vi "JoyStick_Global.vi"() -> ()   [LabVIEW 2015]
doc: "This global VI can contain as many global variables as you need. Place a control on the panel, give it a good name. To read or write to it from a VI, drag the icon to the diagram of that VI. You can also drag from the project. Click on the node to change which global you access. You shouldn't have multiple locations writing to a global or it will cause a race-condition."
uses:
  <vilib>/Rock Robotics/WPI/Camera/WPI_CameraImageSize.ctl
  <vilib>/Rock Robotics/WPI/DriverStation/WPI_DriverStationRobotMode2.ctl
panel:
  out "Intake_Sensor_LED":bool
  out "Stage_Sensor_LED":bool
  out "Light_Show":bool
  out "Low_Goal":bool
  in  "Climb_Speed":dbl
  in  "Climb_Pneu":bool
  in  "Auto_Aim":bool
  in  "Flipper_Man":bool
  in  "Lower_Intake_Def":bool
  in  "Raise_Intake_Def":bool
  in  "Lower_Intake_Arm":bool
  in  "Raise_Intake_Arm":bool
  in  "Stage_Motor_Man":dbl
  in  "Intake_Motor_Man":dbl
  in  "Right_Speed":dbl
  in  "Left_Speed":dbl
  in  "Right_Dist":dbl
  in  "Left_Dist":dbl
  in  "Cheval":bool
  in  "Intake Stage":bool
  out "Speed Toggle":bool
  in  "Intake":bool
  out "Gear_Toggle":bool
  out "Climb":bool
  out "Portcullis":bool
  in  "Right_Joystick_Y":dbl
  in  "Right_Joystick_X":dbl
  in  "Left_Joystick_Y":dbl
  out "Far_Shot":bool
  in  "Left_Joystick_X":dbl
  out "Close_Shot":bool
  in  "Robot Mode":T1
  in  "image size":T2=enum."320x240"
  in  "Enable Vision":bool
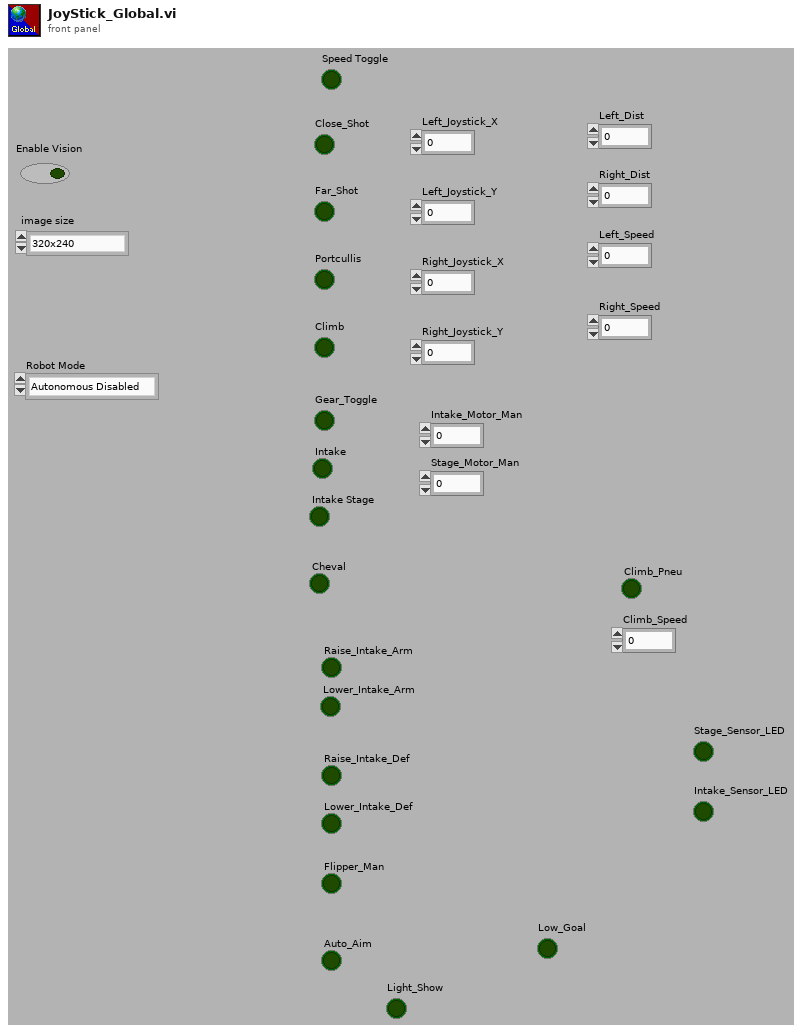
[diagram p1: front panel]
types:
  T1 = typedef "WPI_DriverStationRobotMode2.ctl" = enum16{"Autonomous Disabled", "Autonomous Enabled", "Teleop Disabled", "Teleop Enabled", "Disconnected", "Finish", "Test Disabled", "Test Enabled", "Emergency Stopped"}
  T2 = typedef "WPI_CameraImageSize.ctl" = enum16{"640x480", "320x240", "160x120", "Custom"}
diagram:
